vi "ACT_Limit_Setpoint_Control_PD_Control_M_A.vi"(0 "SI804.lvclass in":refnum<class "SI804.lvclass">, 5 "3 JSA10 DT112 XA01":bool, 7 "3 JSD40 DX101 XA01":bool, 11 "error in":errorcluster) -> (4 "SI804.lvclass out":refnum<class "SI804.lvclass">, 6 "ACT SP Ctrl":bool, 8 "PD-Control M/A":bool, 15 "error out":errorcluster)   [LabVIEW 2022 SP3, in "SI804.lvclass"]
uses:
  SI804.lvclass
  SI804.lvclass/SI804.ctl
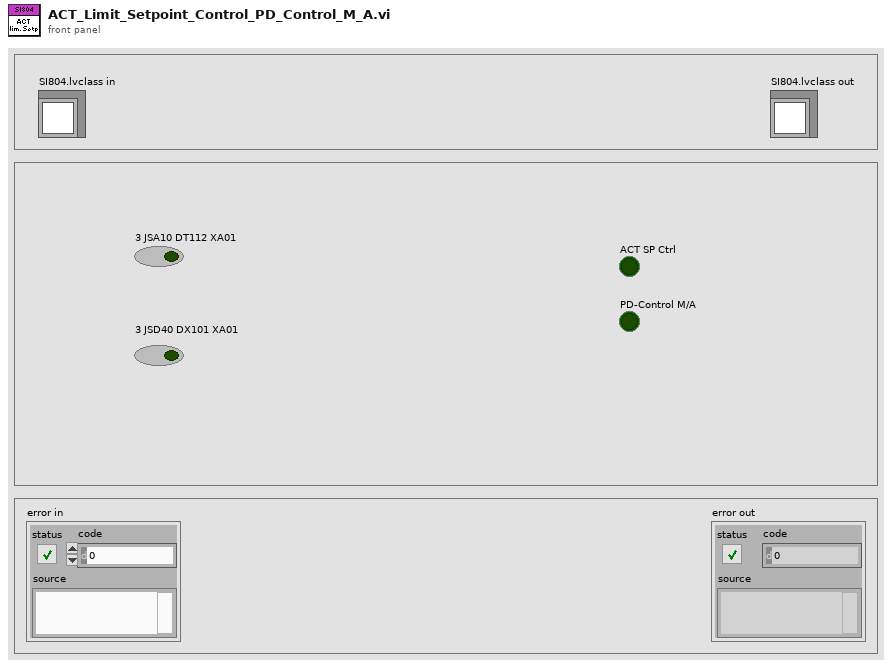
[diagram p1: front panel]
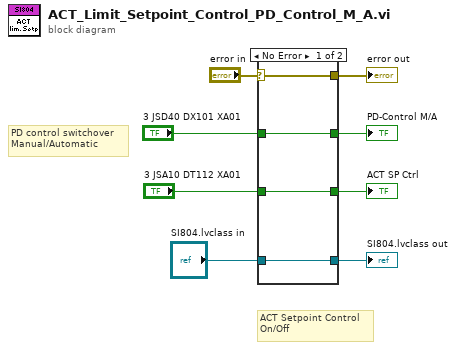
[diagram p0: block diagram]
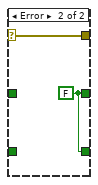
[diagram p2: hidden frame]
diagram:
  # "PD control switchover\nManual/Automatic"
  # "ACT Setpoint Control\nOn/Off"
  n1 = case shown="No Error" "error in" {
    selector: "error in" -> [w10 w13]
    tunnel: "3 JSA10 DT112 XA01" -> [w12 _]
    tunnel: "3 JSD40 DX101 XA01" -> [w11 _]
    tunnel: [w12 w14] -> w5
    tunnel: [w11 w14] -> w4
    tunnel: [w10 w13] -> w3
    tunnel: "SI804.lvclass in" -> [w9 _]
    tunnel: [w9 _] -> w1
    frame No Error {
    }
    frame Error {
      w14 = FALSE ("3 JSA10 DT112 XA01")
    }
  }
  "ACT SP Ctrl" <- w5
  "PD-Control M/A" <- w4
  "error out" <- w3
  "SI804.lvclass out" <- w1
